vi "Config File Ref FGV.vi"(7 "Method":enum16{"Get", "Set"}(ring), 11 "config refnum in":T1) -> (3 "config refnum out":T1)   [LabVIEW 2014]
uses:
  <vilib>/Utility/config.llb/Config Data RefNum.ctl
  <vilib>/Utility/config.llb/NI_LVConfig.lvlib
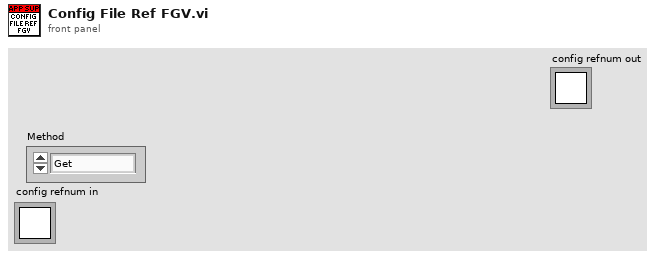
[diagram p1: front panel]
types:
  T1 = typedef "NI_LVConfig.lvlib/Config Data RefNum.ctl" = refnum<k1>
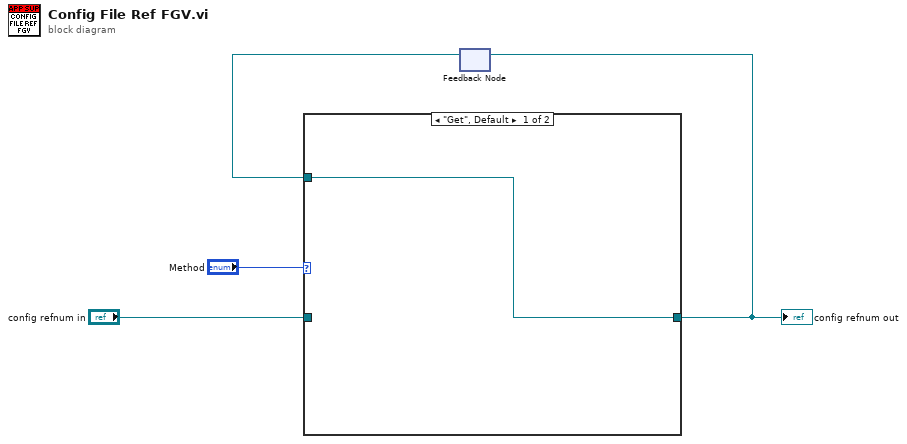
[diagram p0: block diagram]
diagram:
  n1 = feedback #1() -> (w2:T1)  [unwired: 1 in]
  n2 = case shown="\"Get\", Default" "Method" {
    tunnel: "config refnum in" -> [_ w6]
    tunnel: [w5 w6] -> w3
    tunnel: w2 -> [w5 _]
    frame "Get", Default {
    }
    frame "Set" {
    }
  }
  "config refnum out" <- w3
  n3 = feedback-in #1(w3) -> ()
